vi "Get_Orientation.vi"(8 "error in":errorcluster, 11 "camera handle in":u64) -> (0 "error out":errorcluster, 1 "PicamOrientation_":T1=1 items=["Normal", "FlippedHorizontally", "FlippedVertically"], 3 "camera handle out":u64)   [LabVIEW 2014, in "PICam.lvlib"]
doc: "PicamAdcQuality is the set of Analog-to-Digital conversion techniques and quality settings\nfor pixel digitization.\n\nPicamAdcQuality_LowNoise Optimized for the lowest noise.\nPicamAdcQuality_HighCapacity Optimized for sensing high levels of radiation.\nPicamAdcQuality_ElectronMultiplied Provides electron multiplication."
uses:
  PICam.lvlib
  Ctrls/PicamOrientation.ctl
  Picam32.dll
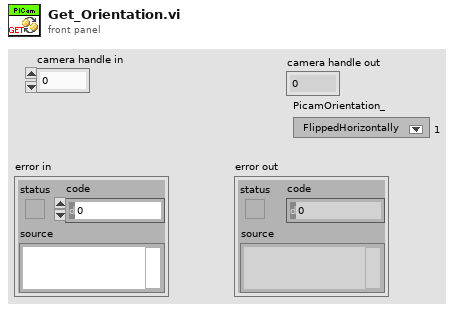
[diagram p1: front panel]
types:
  T1 = typedef "PICam.lvlib/PicamOrientation.ctl" = u32
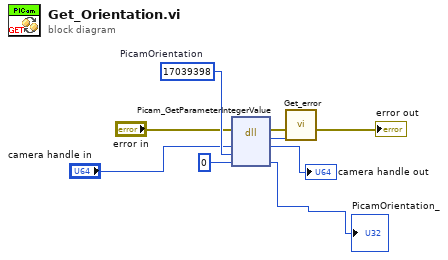
[diagram p0: block diagram]
diagram:
  w5 = u32 17039398  # PicamOrientation
  n1 = dll-call lib="Picam32.dll" fn="Picam_GetParameterIntegerValue"(error in="error in", "camera"="camera handle in", "PicamParameter"=w5, "Orientation"=u32 0 ("AdcAnalogGain")) -> (error out=w9:errorcluster, "return type"=w8:i32, "camera"=→"camera handle out":u64, "Orientation"=→"PicamOrientation_":u32)  [unwired: 3 in, 1 out]
  n2 = call "Get_error.vi"("PICam_Error"=w8, "error in (no error)"=w9) -> ("error out"=→"error out":errorcluster)  [unwired: 9 in]
